vi "Initialize pretomo IMAQ.vi"(8 "error in (no error)":errorcluster, 11 "Tomo in":refnum<class "Tomo.lvclass">) -> (0 "error out":errorcluster, 3 "Tomo out":refnum<class "Tomo.lvclass">)   [LabVIEW 2012, in "Tomo.lvclass"]
uses:
  Tomo.lvclass
  Tomo.lvclass/Tomo.ctl
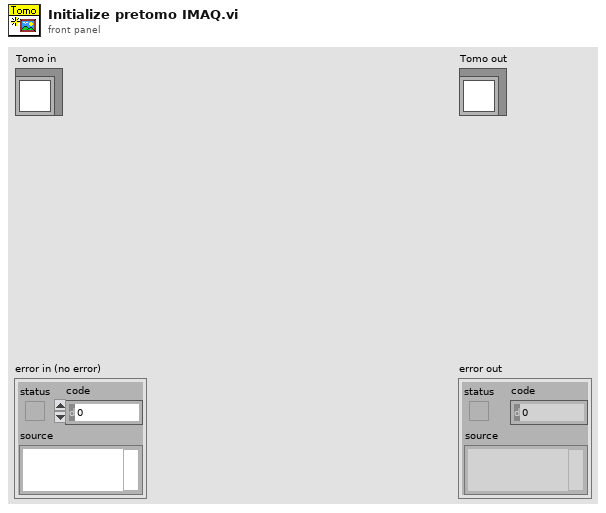
[diagram p1: front panel]
types:
  T1 = typedef "Image Type" = u32
  T2 = typedef "IMAQ Image.ctl" = refnum<image>
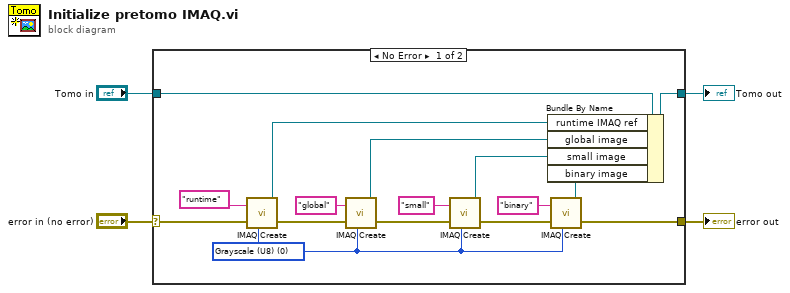
[diagram p0: block diagram]
diagram:
  n1 = case shown="No Error" "error in (no error)" {
    selector: "error in (no error)" -> [w8 w22]
    tunnel: [w18 w22] -> w3
    tunnel: [w16 w21] -> w1
    tunnel: "Tomo in" -> [w17 w21]
    frame No Error {
      w6 = T1 0 items=["Grayscale (U8)", "Grayscale (I16)", "Grayscale (SGL)", "Complex (CSG)", "RGB (U32)", "HSL (U32)", "RGB (U64)", "Grayscale (U16)"] ("Image Type")
      n2 = call "IMAQ Create"("Image Name"="runtime", "Image Type"=w6, "error in (no error)"=w8) -> ("New Image"=w5:T2, "error out"=w7:errorcluster)  [unwired: 2 in]
      n3 = call "IMAQ Create"("Image Name"="global", "Image Type"=w6, "error in (no error)"=w7) -> ("New Image"=w12:T2, "error out"=w20:errorcluster)  [unwired: 2 in]
      n4 = call "IMAQ Create"("Image Name"="small", "Image Type"=w6, "error in (no error)"=w20) -> ("New Image"=w11:T2, "error out"=w19:errorcluster)  [unwired: 2 in]
      n5 = call "IMAQ Create"("Image Name"="binary", "Image Type"=w6, "error in (no error)"=w19) -> ("New Image"=w10:T2, "error out"=w18:errorcluster)  [unwired: 2 in]
      n6 = Bundle By Name(cluster=w17, "runtime IMAQ ref"=w5, "global image"=w12, "small image"=w11, "binary image"=w10) -> (w16:refnum<class "Tomo.lvclass">)
    }
    frame Error {
    }
  }
  "error out" <- w3
  "Tomo out" <- w1
